vi "PIDController_SetPeriod.vi"(8 "Period":dbl, 11 "in PID_CONTROLLER":T1={"Kp"=0.0, "Ki"=0.0, "Kd"=0.0, "Period"=0.0, "Max_Integral"=0.0, "Min_Integral"=0.0, "Max_Input"=0.0, "Min_Input"=0.0, "Continuous"=FALSE, "PositionError"=0.0, "VelocityError"=0.0, "PrevError"=0.0, "TotalError"=0.0, "PositionTolerance"=0.0, "VelocityTolerance"=0.0, "SetPoint"=0.0, "Kf"=0.0, "Prev_Deriv"=0.0, "Prev_Deriv 2"=0.0, "DerivativeFilter"=FALSE, "Min_Output"=-9.99e+35, "Max_Output"=9.9e+35, "Prev_F_P"=0.0, "Prev_F_P_2"=0.0, "AntiWindupActive"=FALSE, "Measurement"=0.0, "IntegralZone"=9.9e+30} {"IntegralZone" format="%16_6e"; "Measurement" format="%16_6e"; "Prev_F_P_2" format="%16_6e"; "Prev_F_P" format="%16_6e"; "Max_Output" format="%16_6e"; "Min_Output" format="%16_6e"; "Prev_Deriv 2" format="%16_6e"; "Prev_Deriv" format="%16_6e"; "Kf" format="%16_6e"; "SetPoint" format="%16_6e"; "VelocityTolerance" format="%16_6e"; "PositionTolerance" format="%16_6e"; "TotalError" format="%16_6e"; "PrevError" format="%16_6e"; "VelocityError" format="%16_6e"; "PositionError" format="%16_6e"; "Min_Input" format="%16_6e"; "Max_Input" format="%16_6e"; "Min_Integral" format="%16_6e"; "Max_Integral" format="%16_6e"; "Period" format="%16_6e"; "Kd" format="%16_6e"; "Ki" format="%16_6e"; "Kp" format="%16_6e"}) -> (3 "out PID_CONTROLLER":T1={"Kp"=0.0, "Ki"=0.0, "Kd"=0.0, "Period"=0.0, "Max_Integral"=0.0, "Min_Integral"=0.0, "Max_Input"=0.0, "Min_Input"=0.0, "Continuous"=FALSE, "PositionError"=0.0, "VelocityError"=0.0, "PrevError"=0.0, "TotalError"=0.0, "PositionTolerance"=0.0, "VelocityTolerance"=0.0, "SetPoint"=0.0, "Kf"=0.0, "Prev_Deriv"=0.0, "Prev_Deriv 2"=0.0, "DerivativeFilter"=FALSE, "Min_Output"=-9.99e+35, "Max_Output"=9.9e+35, "Prev_F_P"=0.0, "Prev_F_P_2"=0.0, "AntiWindupActive"=FALSE, "Measurement"=0.0, "IntegralZone"=9.9e+30} {"IntegralZone" format="%16_6e"; "Measurement" format="%16_6e"; "Prev_F_P_2" format="%16_6e"; "Prev_F_P" format="%16_6e"; "Max_Output" format="%16_6e"; "Min_Output" format="%16_6e"; "Prev_Deriv 2" format="%16_6e"; "Prev_Deriv" format="%16_6e"; "Kf" format="%16_6e"; "SetPoint" format="%16_6e"; "VelocityTolerance" format="%16_6e"; "PositionTolerance" format="%16_6e"; "TotalError" format="%16_6e"; "PrevError" format="%16_6e"; "VelocityError" format="%16_6e"; "PositionError" format="%16_6e"; "Min_Input" format="%16_6e"; "Max_Input" format="%16_6e"; "Min_Integral" format="%16_6e"; "Max_Integral" format="%16_6e"; "Period" format="%16_6e"; "Kd" format="%16_6e"; "Ki" format="%16_6e"; "Kp" format="%16_6e"})   [LabVIEW 2019, in "Trajectory_Library.lvlib"]
doc: "Sets the period, in seconds, of this controller.\n \nInputs:\n - PID_Controller -- PID_Controller data cluster\n - period -- the period of the controller.\n\nOutputs:\n - PID_Controller -- Updated PID_Controller data cluster"
uses:
  Trajectory_Library.lvlib
  TypeDef/PID_CONTROLLER.ctl
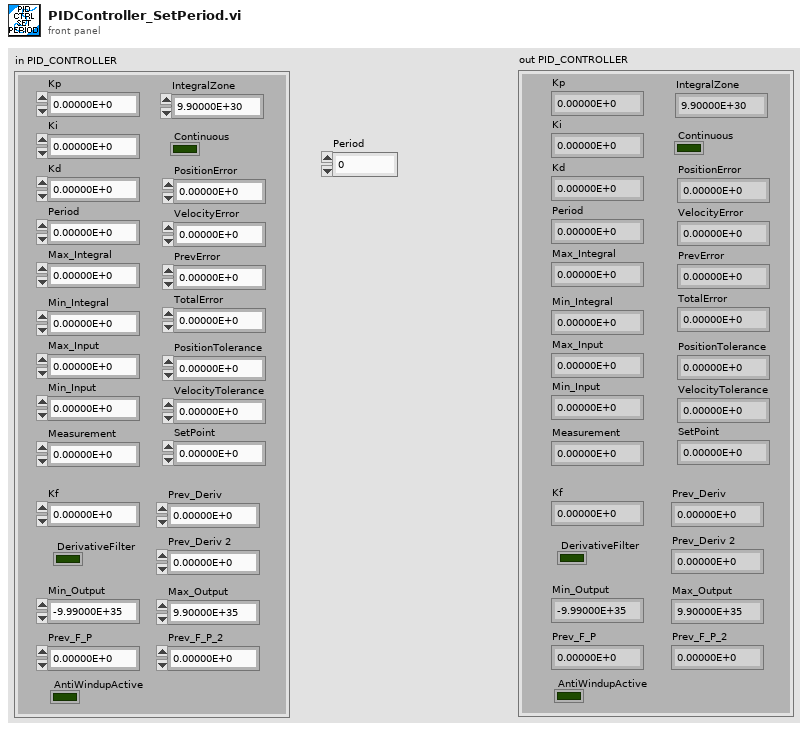
[diagram p1: front panel]
types:
  T1 = typedef "Trajectory_Library.lvlib/PID_CONTROLLER.ctl" = cluster{"Kp":dbl, "Ki":dbl, "Kd":dbl, "Period":dbl, "Max_Integral":dbl, "Min_Integral":dbl, "Max_Input":dbl, "Min_Input":dbl, "Continuous":bool, "PositionError":dbl, "VelocityError":dbl, "PrevError":dbl, "TotalError":dbl, "PositionTolerance":dbl, "VelocityTolerance":dbl, "SetPoint":dbl, "Kf":dbl, "Prev_Deriv":dbl, "Prev_Deriv 2":dbl, "DerivativeFilter":bool, "Min_Output":dbl, "Max_Output":dbl, "Prev_F_P":dbl, "Prev_F_P_2":dbl, "AntiWindupActive":bool, "Measurement":dbl, "IntegralZone":dbl}
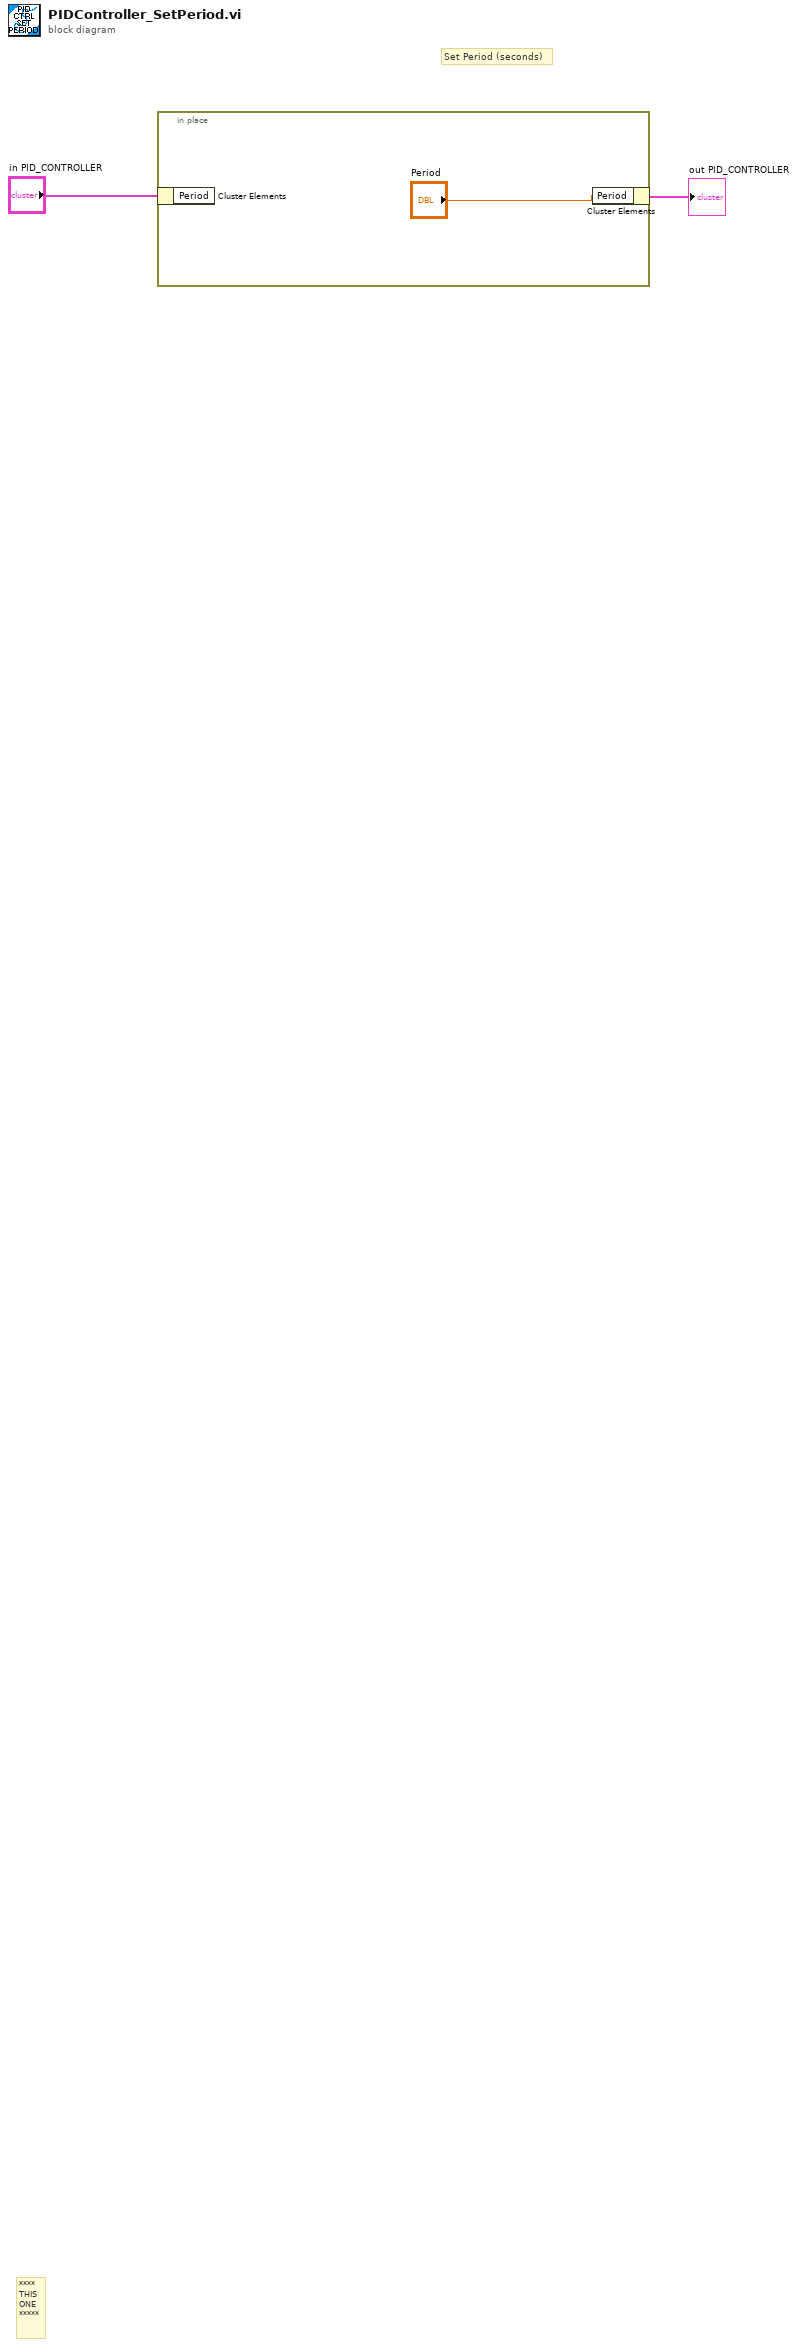
[diagram p0: block diagram]
diagram:
  # "Set Period (seconds)"
  # "****\nTHIS\nONE\n*****"
  n1 = in-place {
    n2 = in-place-cluster #1("in PID_CONTROLLER") -> ()  [unwired: 1 out]
    n3 = in-place-cluster #1("Period"="Period") -> (→"out PID_CONTROLLER":T1)
  }
